vi "ELVIS III v1.0 Unreserve AO Block.vi"(7 "Allow multiple opens?":bool, 8 "error in (no error)":errorcluster, 10 "AO (N Samples) Channel List":T1) -> (0 "error out":errorcluster)   [LabVIEW 2021]
uses:
  <vilib>/myRIO/Common/Instrument Driver Framework/myRIO v1.0/AO Block/typedefs/AO Block Channels List.ctl
  <vilib>/myRIO/Common/Instrument Driver Framework/myRIO v1.0/AO Block/typedefs/AO Block Channels Enum.ctl
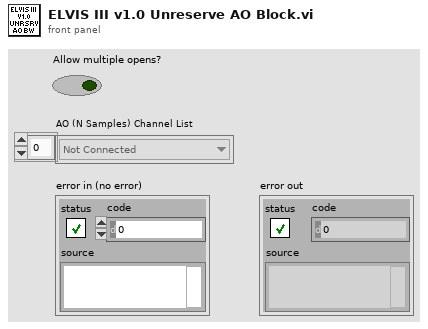
[diagram p1: front panel]
types:
  T1 = typedef "AO Block Channels List.ctl" = T2[]
  T2 = typedef "AO Block Channels Enum.ctl" = enum16{"Not Connected", "A/AO0 (N Samples)", "A/AO1 (N Samples)", "B/AO0 (N Samples)", "B/AO1 (N Samples)"}
  T3 = typedef "ELVIS III v1.0 Channel Reservation List.ctl" = T4[]
  T4 = typedef "ELVIS III v1.0 Channel Reservation Info.ctl" = cluster{"Channel Name":string, "Connector":T5, "MutexIDs":u32[]}
  T5 = typedef "ELVIS III v1.0 Connector List.ctl" = enum32{"None", "ConnectorA", "ConnectorB"}
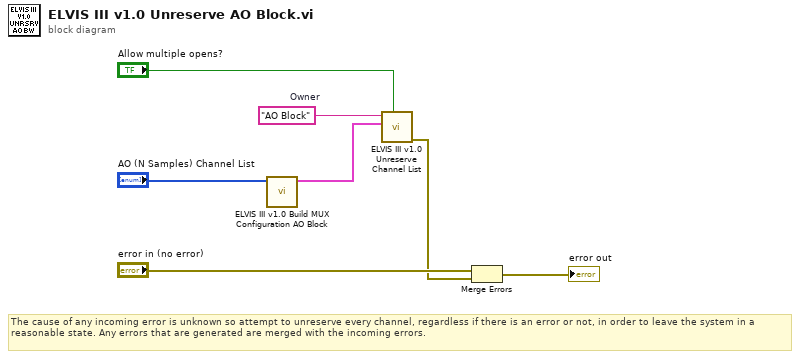
[diagram p0: block diagram]
diagram:
  w2 = "AO Block"  # Owner
  # "The cause of any incoming error is unknown so attempt to unreserve every channel, regardless if there is an error or not, in order to leave the system in a reasonable state. Any errors that are generated are merged with the incoming errors."
  n1 = call <vilib>:"ELVIS III v1.0 Build MUX Configuration AO Block.vi"("AO (N Samples) Channels List"="AO (N Samples) Channel List") -> ("Channel Reservation Info"=w3:T3)  [unwired: 9 in, 1 out]
  n2 = call <vilib>:"ELVIS III v1.0 Unreserve Channel List.vi"("Allow multiple opens?"="Allow multiple opens?", "Channel Reservation List"=w3, "Owner"=w2) -> ("error out"=w1:errorcluster)  [unwired: 8 in]
  n3 = Merge Errors("error in (no error)", w1) -> (→"error out":errorcluster)
